vi "主动发送数据生成Condition(子VI).vi"(7 "结束时间":timestamp, 8 "数据发送协议":enum16{"2005-212协议", "2017-212协议"}(ring)=enum."2017-212协议", 9 "database":string, 10 "Label.Text":string, 11 "数值":i32) -> (0 "date/time string":string, 1 "database溢出":bool, 2 "columns":string[](array[string])=["时间", "测量模式", "数据类型", "检测值", "单位", "数据标识"], 3 "CONDITION":string)   [LabVIEW 2016, in "数据传输系统-03.lvlib"]
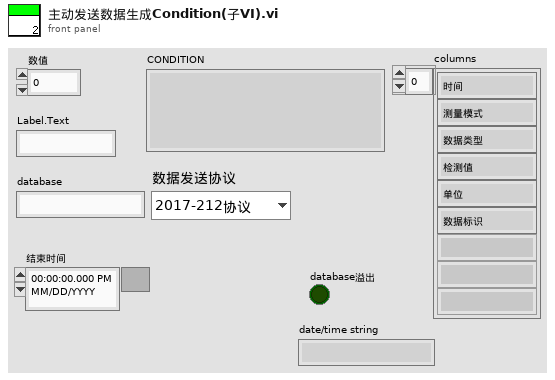
[diagram p1: front panel]
types:
  T1 = cluster{"time1":string, "time2":string, "time3":string, "time4":string, "time5":string, "time6":string, "time7":string, "time8":string, "time9":string, "time10":string, "time11":string, "time12":string, "time13":string, "time14":string, "time15":string, "time16":string, "time17":string, "time18":string, "time19":string, "time20":string, "time21":string, "time22":string, "time23":string, "time24":string, "time25":string, "time26":string, "time27":string, "time28":string, "time29":string, "time30":string, "time31":string, "time32":string, "time33":string, "time34":string, "time35":string, "time36":string, "time37":string}
  T2 = typedef "LVDateTimeRec.ctl" = cluster{"秒数的小数部分":dbl, "秒":i32, "分":i32, "时":i32, "日":i32, "月":i32, "年":i32, "天数（周）":i32, "天数（年）":i32, "DST":i32}
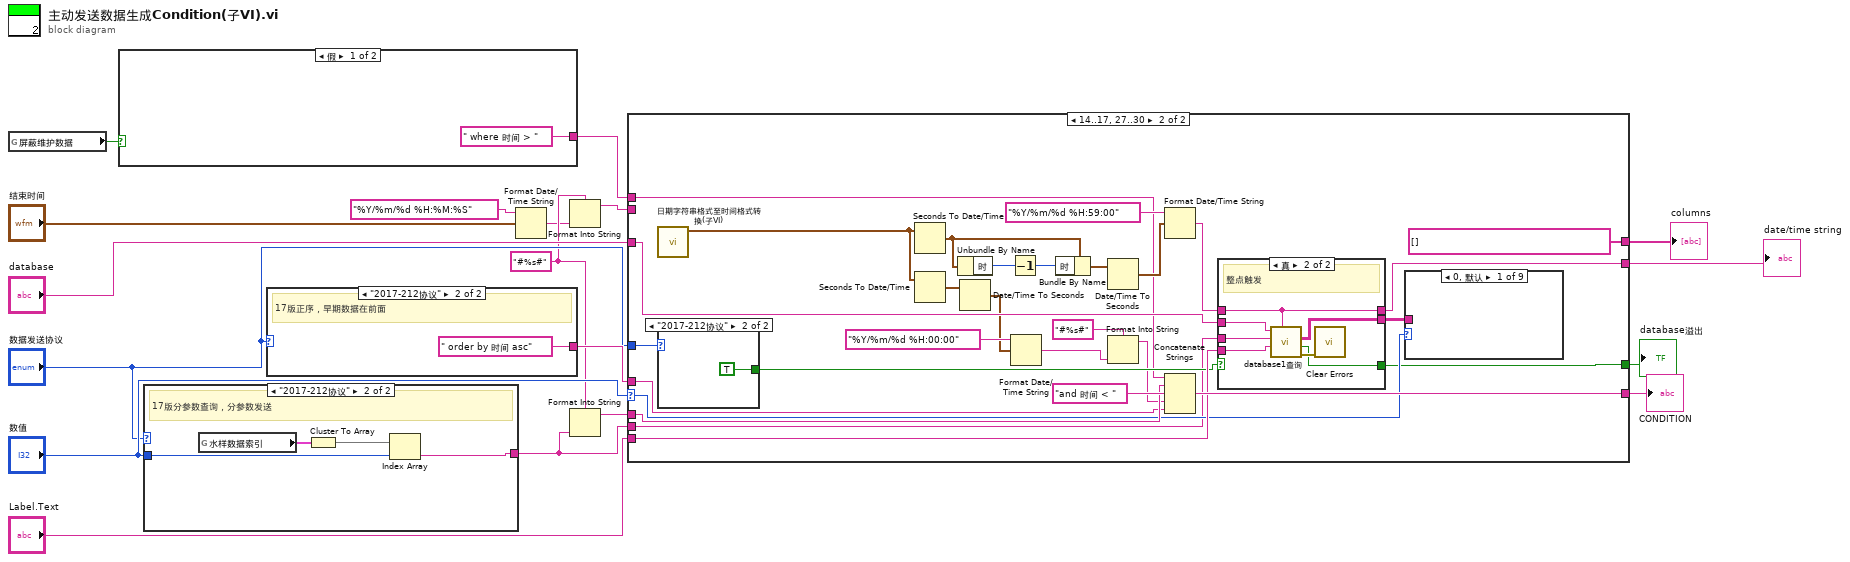
[diagram p0: block diagram]
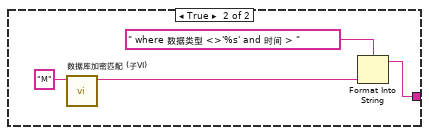
[diagram p2: hidden frame]
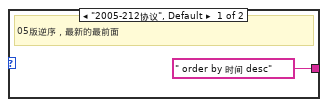
[diagram p3: hidden frame]
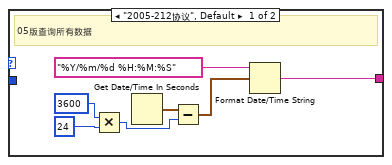
[diagram p4: hidden frame]
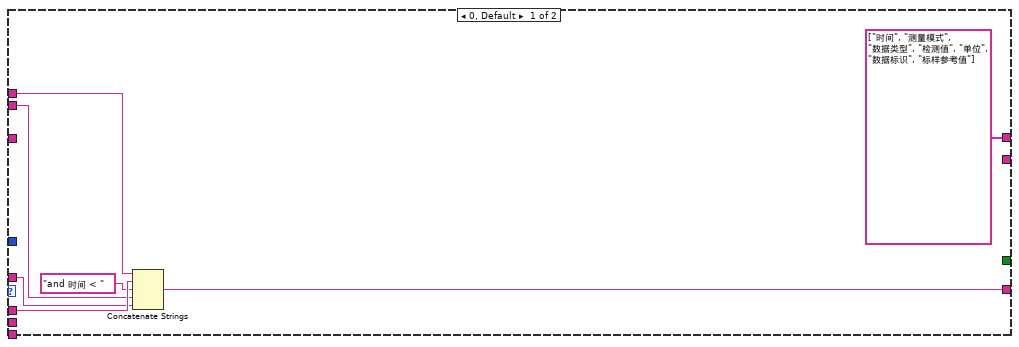
[diagram p5: hidden frame]
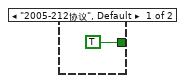
[diagram p6: hidden frame]
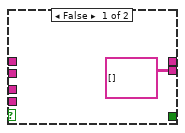
[diagram p7: hidden frame]
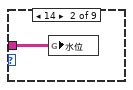
[diagram p8: hidden frame]
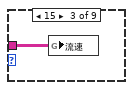
[diagram p9: hidden frame]
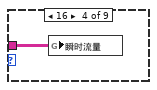
[diagram p10: hidden frame]
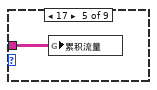
[diagram p11: hidden frame]
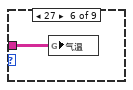
[diagram p12: hidden frame]
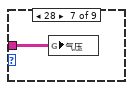
[diagram p13: hidden frame]
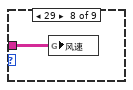
[diagram p14: hidden frame]
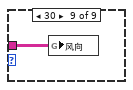
[diagram p15: hidden frame]
diagram:
  w6 = "#%s#" ("初始字符串")
  n1 = global read "断电保存全局.vi" "屏蔽维护数据"() -> (w4:bool)
  n2 = case shown="假" w4 {
    tunnel: [" where 时间 > " w22] -> w5
    frame False {
    }
    frame True {
      n3 = call "数据库加密匹配 (子VI).vi"("输入参数"="M") -> ("Encoded String"=w20:string)  [unwired: 10 in]
      n4 = Format Into String(format string=" where 数据类型 <>'%s' and 时间 > ", w20) -> (resulting string=w22:string)  [unwired: 2 in, 1 out]
    }
  }
  n5 = case shown="\"2017-212协议\"" "数据发送协议" {
    tunnel: [w29 w31] -> w18
    tunnel: "数值" -> [_ w32]
    frame "2005-212协议", Default {
      # "05版查询所有数据"
      n6 = Multiply(x=3600, y=24) -> (x*y=w24:i32)
      n7 = Get Date/Time In Seconds() -> (seconds since 1Jan1904=w28:timestamp)
      n8 = Subtract(x=w28, y=w24) -> (x-y=w27:timestamp)
      n9 = Format Date/Time String(time format string (%c)="%Y/%m/%d %H:%M:%S" ("时间格式字符串(%c)"), seconds (now)=w27) -> (date/time string=w29:string)  [unwired: 1 in]
    }
    frame "2017-212协议" {
      # "17版分参数查询，分参数发送"
      n10 = global read "全局 水样时间.vi" "水样数据索引"() -> (w33:T1)
      n11 = Cluster To Array(cluster=w33) -> (array=w34:string[])
      n12 = Index Array(array=w34, index=w32) -> (element=w31:string)
    }
  }
  n13 = case shown="\"2017-212协议\"" "数据发送协议" {
    tunnel: [" order by 时间 desc" ("字符串") " order by 时间 asc" ("字符串")] -> w12
    frame "2005-212协议", Default {
      # "05版逆序，最新的最前面"
    }
    frame "2017-212协议" {
      # "17版正序，早期数据在前面"
    }
  }
  n14 = Format Date/Time String(time format string (%c)="%Y/%m/%d %H:%M:%S" ("时间格式字符串(%c)"), seconds (now)="结束时间") -> (date/time string=w3:string)  [unwired: 1 in]
  n15 = Format Into String(format string=w6, w3) -> (resulting string=w14:string)  [unwired: 2 in, 1 out]
  n16 = Format Into String(format string=w6, w18) -> (resulting string=w13:string)  [unwired: 2 in, 1 out]
  n17 = case shown="14..17, 27..30" "数值" {
    selector: "数值" -> [_ w66]
    tunnel: w13 -> [w43 w70]
    tunnel: [w42 w71] -> w8
    tunnel: w14 -> [w40 _]
    tunnel: "database" -> [_ w69]
    tunnel: "Label.Text" -> [_ w68]
    tunnel: w18 -> [_ w54]
    tunnel: w12 -> [w39 w65]
    tunnel: [string[] ["时间", "测量模式", "数据类型", "检测值", "单位", "数据标识", "标样参考值"] ("columns") string[] [] ("columns")] -> w11
    tunnel: "数据发送协议" -> [_ w62]
    tunnel: w5 -> [w37 w53]
    tunnel: [_ w45] -> w1
    tunnel: [_ w44] -> w2
    frame 0, Default {
      n18 = Concatenate Strings(w37, w43, "and 时间 < " ("字符串"), w40, w39) -> (w42:string)
    }
    frame 14..17, 27..30 {
      n19 = call "日期字符串格式至时间格式转换(子VI).vi"() -> ("time stamp"=w50:timestamp)  [unwired: 11 in]
      n20 = case shown="\"2017-212协议\"" w62 {
        tunnel: [TRUE TRUE] -> w64
        frame "2005-212协议", Default {
        }
        frame "2017-212协议" {
        }
      }
      n21 = Seconds To Date/Time(time stamp (now)=w50) -> (date time rec=w59:T2)  [unwired: 1 in]
      n22 = Seconds To Date/Time(time stamp (now)=w50) -> (date time rec=w49:T2)  [unwired: 1 in]
      n23 = Unbundle By Name(w59) -> ("时"=w60:i32)
      n24 = Date/Time To Seconds(2:w49) -> (0:w51:timestamp)  [unwired: 1 in]
      n25 = Decrement(x=w60) -> (x-1=w61:i32)
      n26 = Format Date/Time String(time format string (%c)="%Y/%m/%d %H:00:00" ("时间格式字符串(%c)"), seconds (now)=w51) -> (date/time string=w47:string)  [unwired: 1 in]
      n27 = Bundle By Name(cluster=w59, "时"=w61) -> (w58:T2)
      n28 = Date/Time To Seconds(2:w58) -> (0:w57:timestamp)  [unwired: 1 in]
      n29 = Format Into String(format string="#%s#" ("初始字符串"), w47) -> (resulting string=w46:string)  [unwired: 2 in, 1 out]
      n30 = Format Date/Time String(time format string (%c)="%Y/%m/%d %H:59:00" ("时间格式字符串(%c)"), seconds (now)=w57) -> (date/time string=w55:string)  [unwired: 1 in]
      n31 = Concatenate Strings(w53, w70, "and 时间 < " ("字符串"), w46, w65) -> (w71:string)
      n32 = case shown="真" w64 {
        tunnel: w69 -> [_ w82]
        tunnel: w68 -> [_ w81]
        tunnel: [string[][] [] ("data") w80] -> w67
        tunnel: w55 -> [_ w77]
        tunnel: w54 -> [_ w78]
        tunnel: [_ w77] -> w45
        tunnel: [_ w76] -> w44
        frame False {
        }
        frame True {
          # "整点触发"
          n33 = call "database1查询.vi"("时间2"=w77, "table"=w81, "时间1"=w78, "database"=w82) -> ("error out"=w79:errorcluster, "database溢出"=w76:bool, "data"=w80:string[][])  [unwired: 3 in, 1 out]
          n34 = call <vilib>:"Clear Errors.vi"("error in (no error)"=w79) -> ()  [unwired: 5 in, 2 out]
        }
      }
      n35 = case shown="0, 默认" w66 {
        tunnel: w67 -> [_ w83 w84 w85 w86 w87 w88 w89 w90]
        frame 0, Default {
        }
        frame 14 {
          n36 = global write "全局 所有参数.vi" "水位"(w83) -> ()
        }
        frame 15 {
          n37 = global write "全局 所有参数.vi" "流速"(w84) -> ()
        }
        frame 16 {
          n38 = global write "全局 所有参数.vi" "瞬时流量"(w85) -> ()
        }
        frame 17 {
          n39 = global write "全局 所有参数.vi" "累积流量"(w86) -> ()
        }
        frame 27 {
          n40 = global write "全局 所有参数.vi" "气温"(w87) -> ()
        }
        frame 28 {
          n41 = global write "全局 所有参数.vi" "气压"(w88) -> ()
        }
        frame 29 {
          n42 = global write "全局 所有参数.vi" "风速"(w89) -> ()
        }
        frame 30 {
          n43 = global write "全局 所有参数.vi" "风向"(w90) -> ()
        }
      }
    }
  }
  "CONDITION" <- w8
  "columns" <- w11
  "database溢出" <- w2
  "date/time string" <- w1
